vi "Button Counter.vi"() -> ()   [LabVIEW 2020]
panel:
  in  "Reset":bool
  out "Time between Presses (s)":dbl
  out "Times Pressed":u32
  in  "Boolean":bool
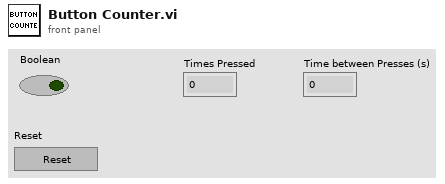
[diagram p1: front panel]
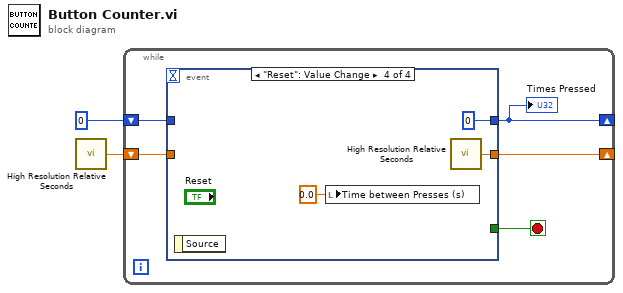
[diagram p0: block diagram]
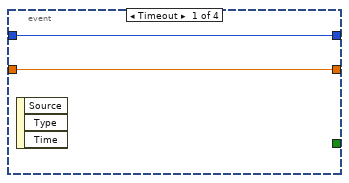
[diagram p2: hidden frame]
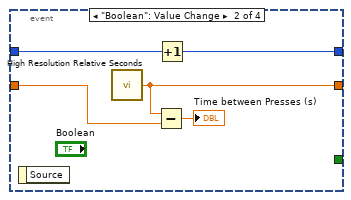
[diagram p3: hidden frame]
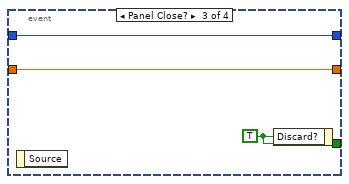
[diagram p4: hidden frame]
diagram:
  n1 = call <vilib>:"High Resolution Relative Seconds.vi"() -> ("relative seconds"=w1:dbl)
  n2 = while {
    shift-right: [w6] -> _
    shift-left: u32 0 ("Times Pressed") -> [w7]
    shift-right: [w3] -> _
    shift-left: w1 -> [w5]
    stop <- w4 stop-if-true
    n3 = event shown="[3] \"Reset\": Value Change" {
      selector: _ -> [_ _ _ _]
      dyn-events: _ -> [_ _ _ _]
      timeout: _ -> [_ _ _ _]
      tunnel: [w9 w13 w17 u32 0 ("Times Pressed")] -> w6
      tunnel: w7 -> [w9 w14 w17 _]
      tunnel: [w8 w11 w16 w19] -> w3
      tunnel: w5 -> [w8 w12 w16 _]
      tunnel: [_ _ w15 _] -> w4
      event Timeout {
        n4 = event-data() -> ()  [unwired: 1 in, 3 out]
      }
      event "Boolean": Value Change {
        n5 = event-data() -> ()  [unwired: 1 in, 1 out]
        n6 = call <vilib>:"High Resolution Relative Seconds.vi"() -> ("relative seconds"=w11:dbl)
        n7 = Subtract(x=w11, y=w12) -> (x-y=→"Time between Presses (s)":dbl)
        n8 = Increment(x=w14) -> (x+1=w13:u32)
      }
      event Panel Close? {
        w15 = TRUE ("Discard?")
        n9 = event-data() -> ()  [unwired: 1 in, 1 out]
        n10 = event-data("Discard?"=w15) -> ()  [unwired: 1 in, 1 out]
      }
      event "Reset": Value Change {
        n11 = event-data() -> ()  [unwired: 1 in, 1 out]
        n12 = local write "Time between Presses (s)"(0.0 ("Time between Presses (s)")) -> ()
        n13 = call <vilib>:"High Resolution Relative Seconds.vi"() -> ("relative seconds"=w19:dbl)
      }
    }
    "Times Pressed" <- w6
  }
